vi "LabVIEW script for delivery of LED light pulses and recoding.vi"() -> ()   [LabVIEW 2013]
uses:
  <vilib>/DAQmx/write.llb/DAQmx Write (Digital Bool 1Line 1Point).vi
  <vilib>/DAQmx/create/channels.llb/DAQmx Create Channel (DO-Digital Output).vi
  <vilib>/vision/driver/Vision Acquisition Express Utility VIs.llb/Vision Acquisition Path Convert (Path).vi
  <vilib>/DAQmx/miscellaneous.llb/DAQmx Fill In Error Info.vi
panel:
  in  "LED ON Frame":i32=150
  out "波形チャート":u32(graph)
  in  "Save movies":bool
  out "Progression indicator":u8(slide)=100 scale=0.0..100.0
  out "loop end":bool=TRUE
  in  "Total frames (30 fps)":i32=300
  in  "Image Logging Path":path=path "C:/mov/test_mov"
  out "Image number":u32=299 caption="Image Number"
  out "Frame rate":dbl=60.0 caption="Frame Rate"
  in  "Stop (F)":bool
  out "Image Out":T1(plugin-control)
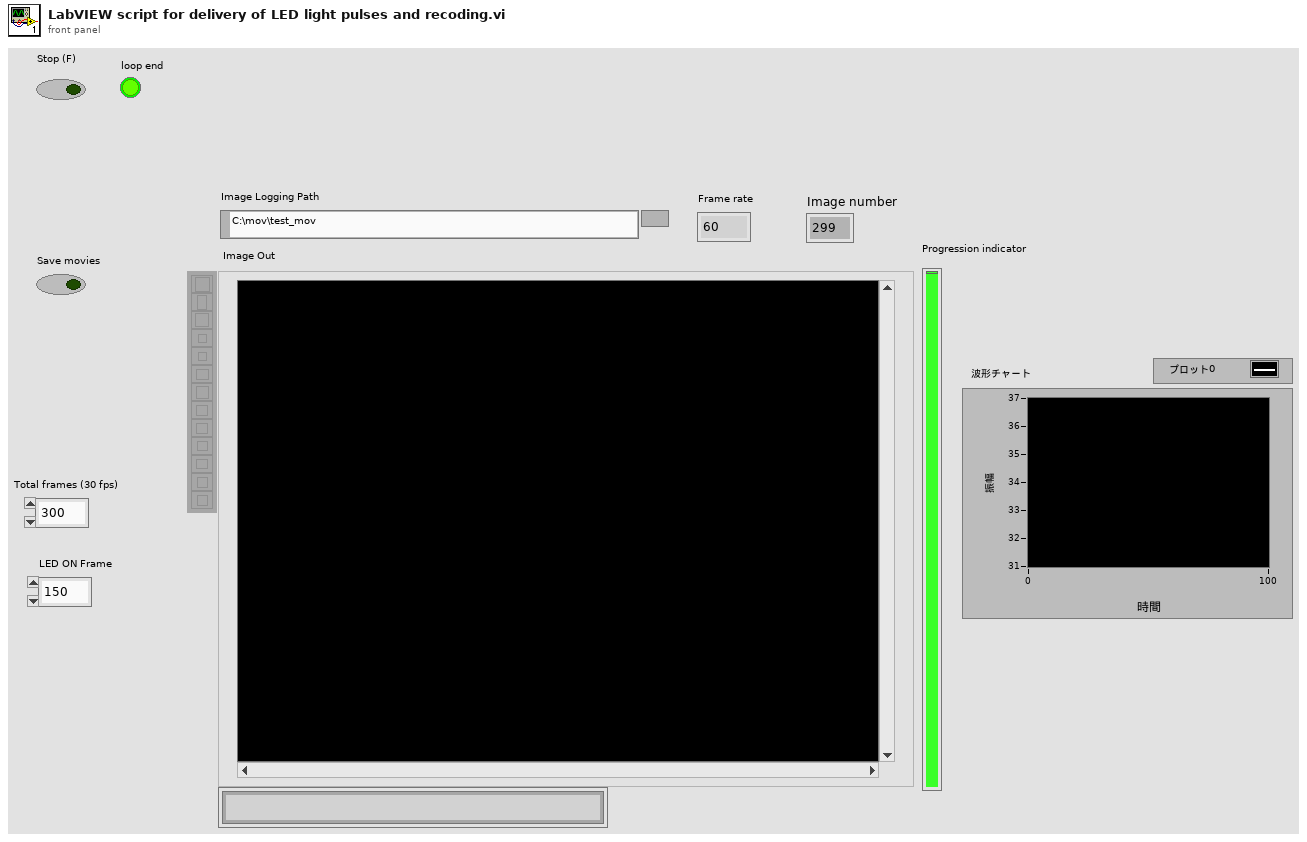
[diagram p1: front panel]
types:
  T1 = typedef "IMAQ Image.ctl" = refnum<image>
  T2 = cluster{"File Type":string, "Quality":u32, "Compress":bool, "Lossless":bool, "Ratio":sgl, "Codec":string, "Frame Rate":u32, "Limit Frames":bool, "Max Frames":u32}
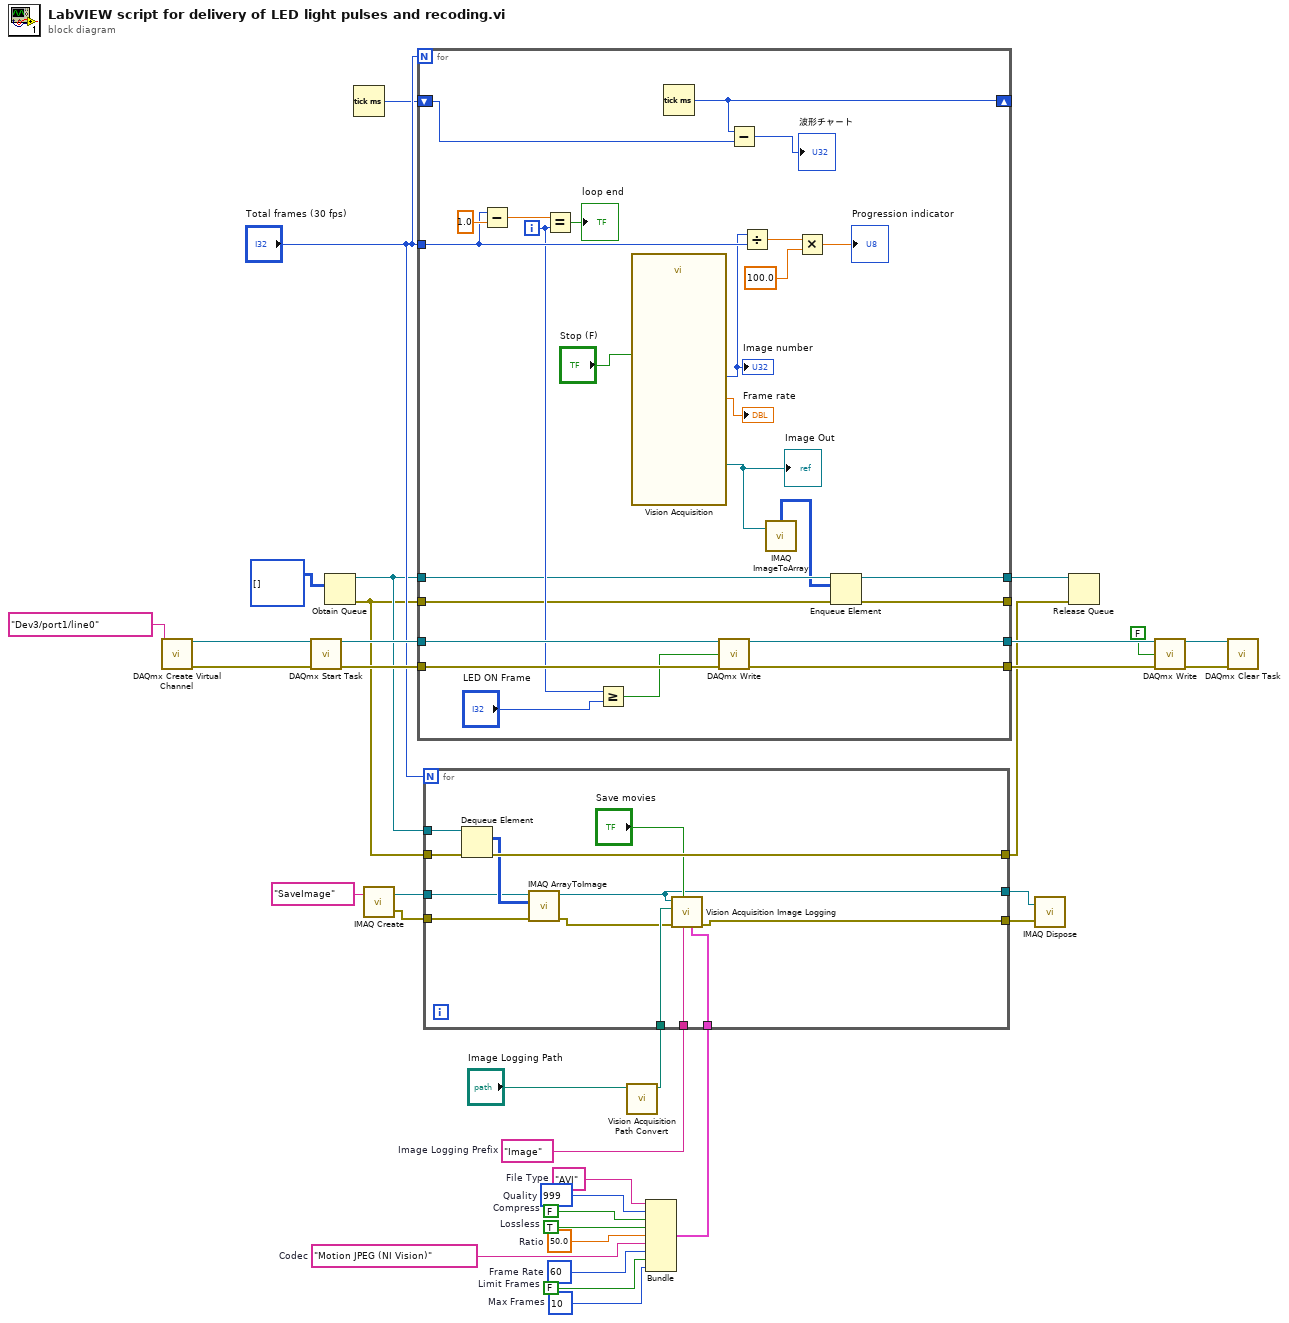
[diagram p0: block diagram]
diagram:
  w9 = "Image"  # Image Logging Prefix
  w15 = sgl 50.0  # Ratio
  w16 = TRUE  # Lossless
  w17 = FALSE  # Compress
  w18 = u32 999  # Quality
  w14 = "Motion JPEG (NI Vision)"  # Codec
  w13 = u32 60  # Frame Rate
  w11 = u32 10  # Max Frames
  w12 = FALSE  # Limit Frames
  w19 = "AVI"  # File Type
  n1 = call-poly <vilib>:"DAQmx Create Virtual Channel.vi"("lines"=tag "Dev3/port1/line0") -> ("task out"=w35:refnum<k21>, "error out"=w34:errorcluster)  [unwired: 13 in]
  n2 = call <vilib>:"DAQmx Start Task.vi"("task/channels in"=w35, "error in"=w34) -> ("task out"=w33:refnum<k21>, "error out"=w32:errorcluster)  [unwired: 12 in]
  n3 = Obtain Queue(element data type=u8[][] [] ("Image Pixels (U8)")) -> (queue out=w22:refnum<queue>, error out=w21:errorcluster)  [unwired: 4 in, 1 out]
  n4 = Tick Count (ms)() -> (millisecond timer value=w1:u32)
  n5 = call "IMAQ Create"("Image Name"="SaveImage") -> ("New Image"=w7:T1, "error out"=w5:errorcluster)  [unwired: 4 in]
  n6 = for {
    N: "Total frames (30 fps)" -> [_]
    tunnel: "Total frames (30 fps)" -> [w58]
    tunnel: w33 -> [w54]
    tunnel: w32 -> [w53]
    tunnel: [w52] -> w30
    tunnel: [w51] -> w29
    tunnel: w22 -> [w44]
    tunnel: [w43] -> w24
    tunnel: [w42] -> _
    tunnel: w21 -> [w41]
    shift-right: [w38] -> _
    shift-left: w1 -> [w37]
    i -> [w50]
    n7 = Subtract(x=w58, y=1.0) -> (x-y=w60:dbl)
    n8 = Equal?(x=w60, y=w50) -> (x = y?=→"loop end":bool)
    n9 = Greater Or Equal?(x=w50, y="LED ON Frame") -> (x >= y?=w48:bool)
    n10 = call "Vision Acquisition"("Stop (F)"="Stop (F)") -> ("Image Out"=w40:T1, "Image Number"=w46:u32, "Frame Rate"=→"Frame rate":dbl)  [unwired: 22 in, 2 out]
    "Image Out" <- w40
    "Image number" <- w46
    n11 = Tick Count (ms)() -> (millisecond timer value=w38:u32)
    n12 = call-poly <vilib>:"DAQmx Write.vi"("task/channels in"=w54, "data"=w48, "error in"=w53) -> ("task out"=w52:refnum<k21>, "error out"=w51:errorcluster)  [unwired: 10 in, 1 out]
    n13 = Subtract(x=w38, y=w37) -> (x-y=→"波形チャート":u32)
    n14 = Divide(x=w46, y=w58) -> (x/y=w57:dbl)
    n15 = call "IMAQ ImageToArray"("Image"=w40) -> ("Image Pixels (U8)"=w39:u8[][])  [unwired: 3 in, 4 out]
    n16 = Multiply(x=w57, y=100.0) -> (x*y=→"Progression indicator":dbl)
    n17 = Enqueue Element(queue=w44, element=w39, error in (no error)=w41) -> (queue out=w43:refnum<queue>, error out=w42:errorcluster)  [unwired: 1 in, 1 out]
  }
  n18 = call-poly <vilib>:"Vision Acquisition Path Convert.vi"("Path In"="Image Logging Path") -> ("Path Out"=w10:path)  [unwired: 10 in]
  n19 = Bundle("File Type"=w19, "Quality"=w18, "Compress"=w17, "Lossless"=w16, "Ratio"=w15, "Codec"=w14, "Frame Rate"=w13, "Limit Frames"=w12, "Max Frames"=w11) -> (w8:T2)  [unwired: 1 out]
  n20 = for {
    N: "Total frames (30 fps)" -> [_]
    tunnel: w22 -> [w74]
    tunnel: w21 -> [w73]
    tunnel: [w72] -> w20
    tunnel: w10 -> [w70]
    tunnel: w9 -> [w69]
    tunnel: w8 -> [w68]
    tunnel: w7 -> [w66]
    tunnel: w5 -> [w65]
    tunnel: [w63] -> w4
    tunnel: [w62] -> w3
    n21 = Dequeue Element(queue=w74, error in (no error)=w73) -> (element=w71:u8[][], error out=w72:errorcluster)  [unwired: 1 in, 2 out]
    n22 = call "IMAQ ArrayToImage"("error in (no error)"=w65, "Image Pixels (U8)"=w71, "Image"=w66) -> ("error out"=w64:errorcluster, "Image Out"=w63:T1)  [unwired: 7 in]
    n23 = call <vilib>:"Vision Acquisition Image Logging.vi"("File Settings"=w68, "Log Image"="Save movies", "error in (no error)"=w64, "Image Logging Prefix"=w69, "Image Logging Path"=w70, "Image In"=w63) -> ("error out"=w62:errorcluster)  [unwired: 1 in, 4 out]
  }
  n24 = call "IMAQ Dispose"("Image"=w4, "error in (no error)"=w3) -> ()  [unwired: 4 in, 1 out]
  n25 = Release Queue(queue=w24, error in (no error)=w20) -> ()  [unwired: 1 in, 3 out]
  n26 = call-poly <vilib>:"DAQmx Write.vi"("task/channels in"=w30, "data"=FALSE, "error in"=w29) -> ("task out"=w27:refnum<k21>, "error out"=w28:errorcluster)  [unwired: 10 in, 1 out]
  n27 = call <vilib>:"DAQmx Clear Task.vi"("task in"=w27, "error in"=w28) -> ()  [unwired: 13 in, 1 out]
